vi "Create Instrument SMO Name.vi"(8 "error in (no error)":errorcluster, 11 "VNA":refnum<class "VNA.lvclass">) -> (0 "error out":errorcluster, 2 "SMO Name":string, 3 "VNA out":refnum<class "VNA.lvclass">)   [LabVIEW 2016, in "VNA.lvclass"]
uses:
  VNA.lvclass
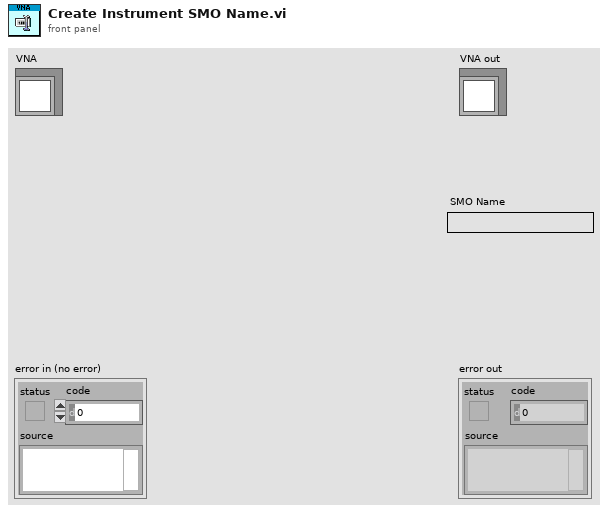
[diagram p1: front panel]
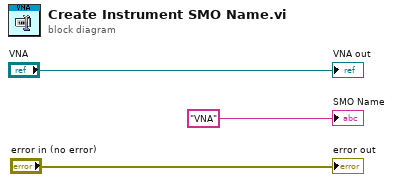
[diagram p0: block diagram]
diagram:
  "error out" <- "error in (no error)"
  "VNA out" <- "VNA"
  "SMO Name" <- "VNA"
